vi "Load Instrument Classes.vi"(8 "error in (no error)":errorcluster, 11 "Control Experiment":refnum<class "SMO.Control Experiment.lvclass">) -> (0 "error out":errorcluster, 3 "Control Experiment out":refnum<class "SMO.Control Experiment.lvclass">)   [LabVIEW 2019, in "SMO.Control Experiment.lvclass"]
uses:
  SMO.Control Experiment.lvclass
  SMO.Control Experiment.lvclass/SMO.Control Experiment.ctl
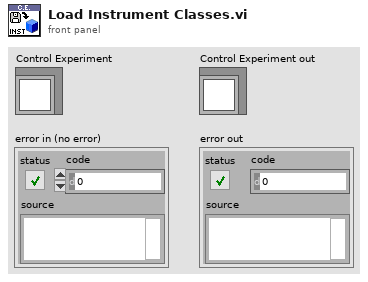
[diagram p1: front panel]
types:
  T1 = typedef "SMO.Control Experiment.lvclass/Instrument--enum.ctl" = enum16{"----- AFM/EBL -----", "AGILENT", "CYPHER", "Gemini2", "JEOL", "MFP3D", "----- Cryostat -----", "CF900", "DR200", "MNK", "PPMS 1", "PPMS 2", "PPMS 3", "----- Optics -----", "THz 1", "THz 2"}
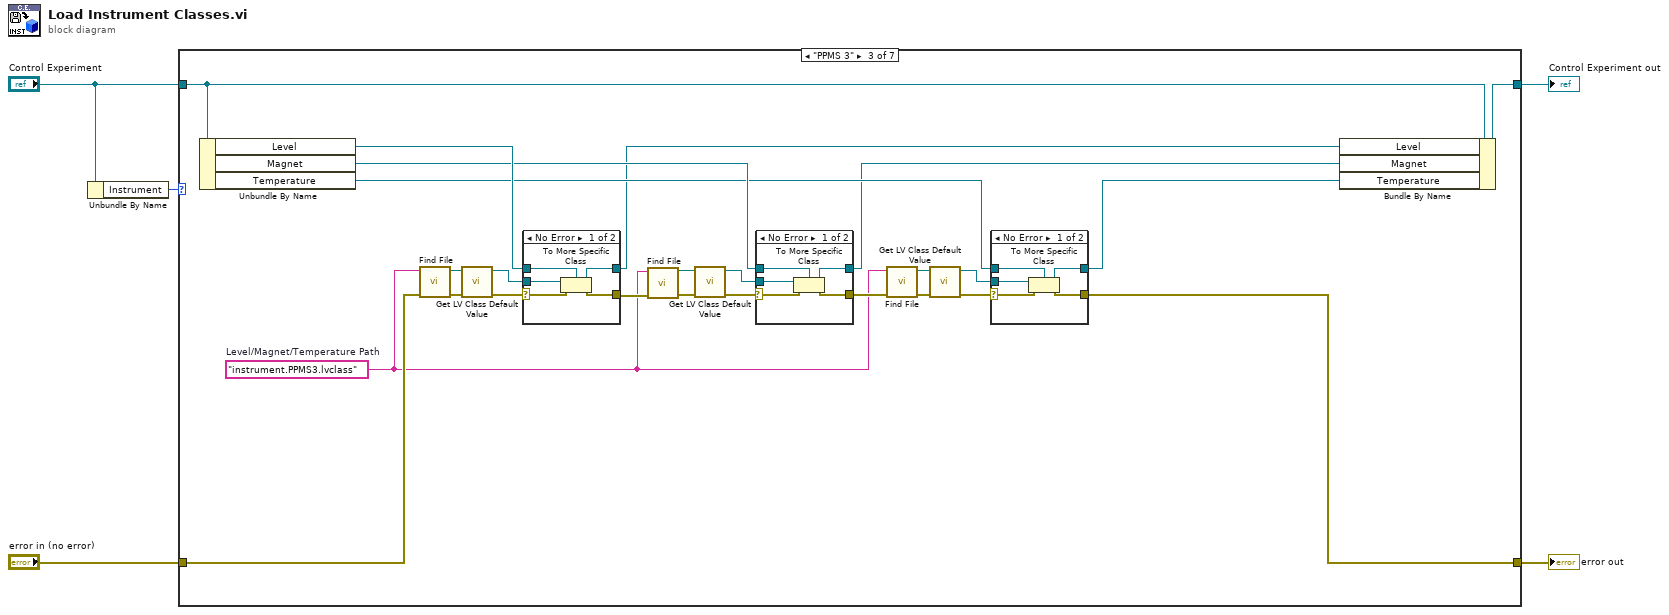
[diagram p0: block diagram]
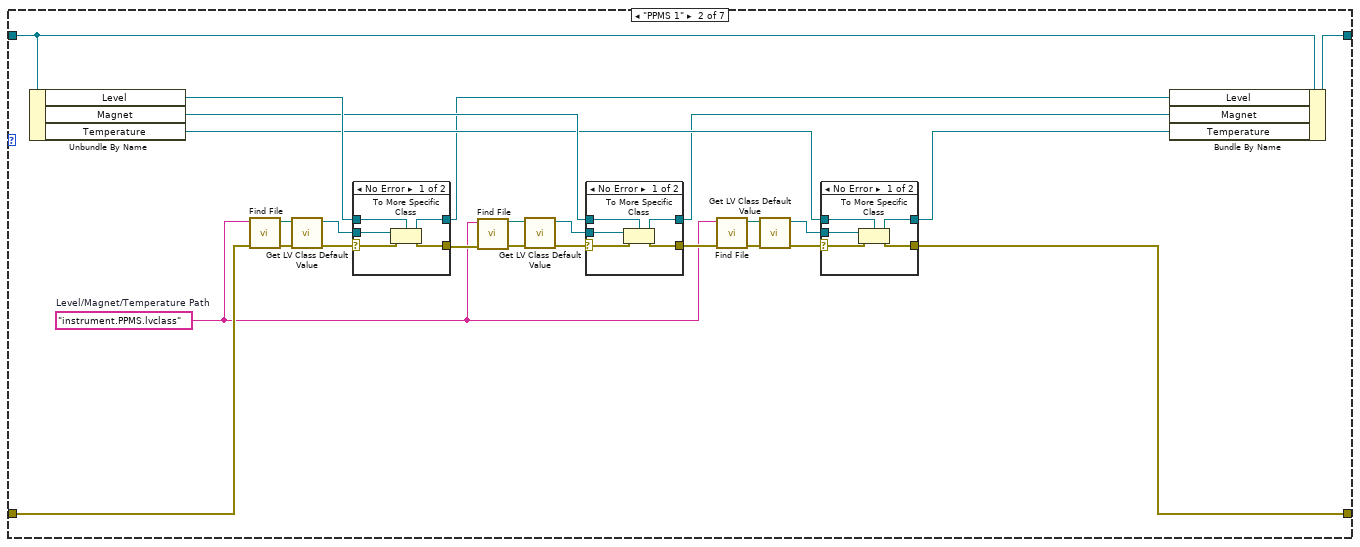
[diagram p3: hidden frame]
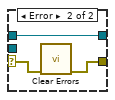
[diagram p4: hidden frame]
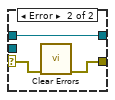
[diagram p5: hidden frame]
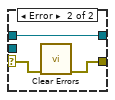
[diagram p6: hidden frame]
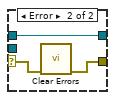
[diagram p7: hidden frame]
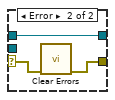
[diagram p8: hidden frame]
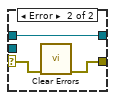
[diagram p9: hidden frame]
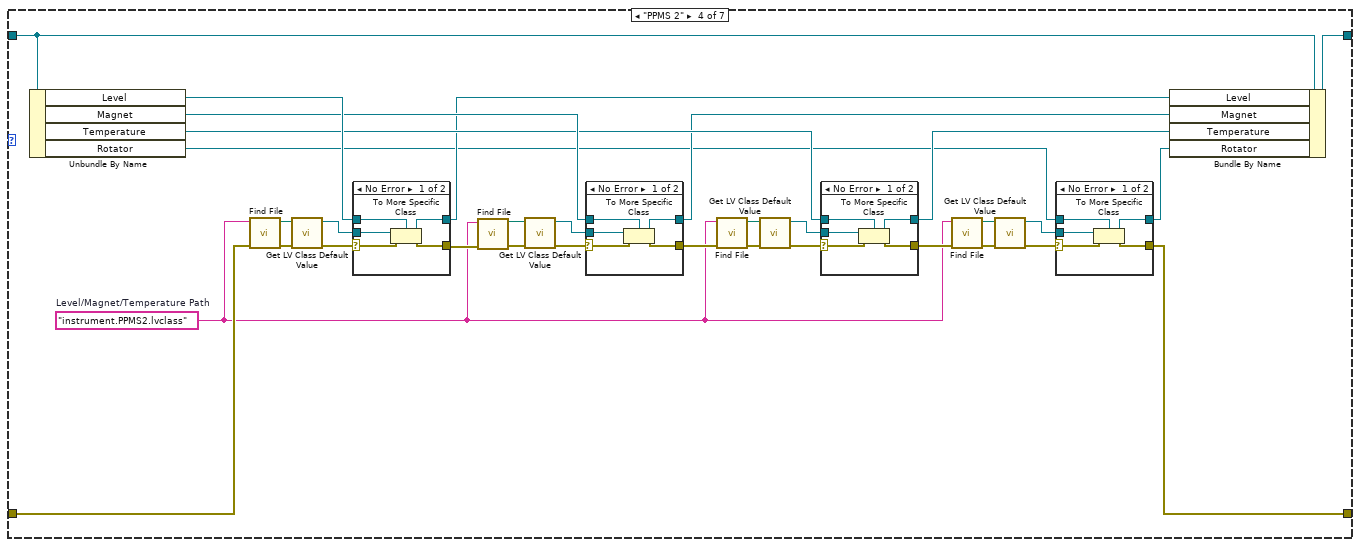
[diagram p10: hidden frame]
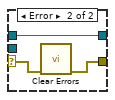
[diagram p11: hidden frame]
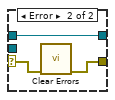
[diagram p12: hidden frame]
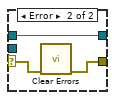
[diagram p13: hidden frame]
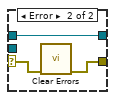
[diagram p14: hidden frame]
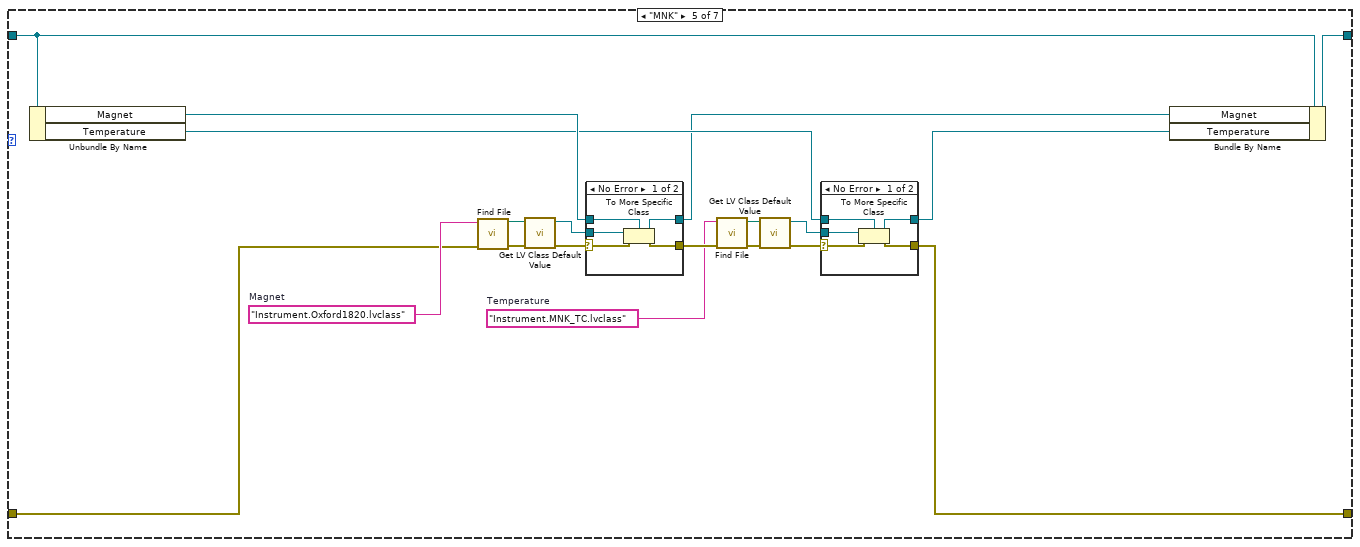
[diagram p15: hidden frame]
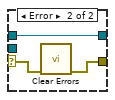
[diagram p16: hidden frame]
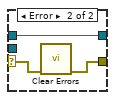
[diagram p17: hidden frame]
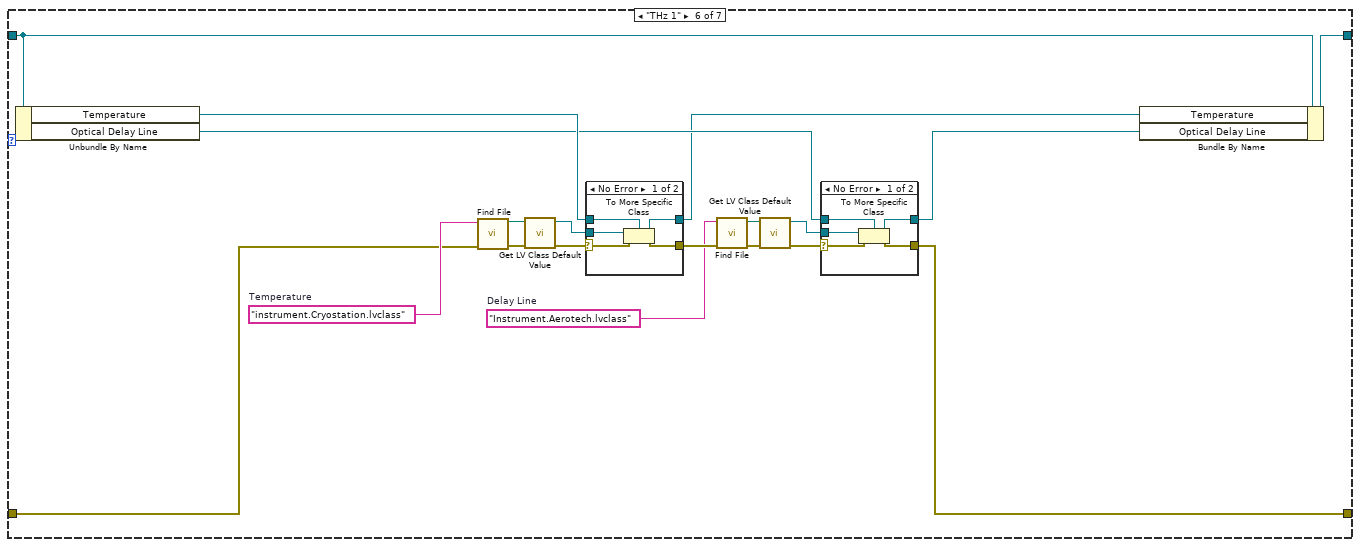
[diagram p18: hidden frame]
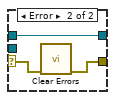
[diagram p19: hidden frame]
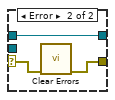
[diagram p20: hidden frame]
diagram:
  n1 = Unbundle By Name("Control Experiment") -> ("Instrument"=w2:T1)
  n2 = case shown="\"PPMS 3\"" w2 {
    tunnel: [w6 w18 w67 w107 w170 w205 w240] -> w5
    tunnel: [w7 w32 w81 w137 w188 w223 w266] -> w4
    tunnel: "Control Experiment" -> [w7 w31 w80 w136 w187 w222 w265]
    tunnel: "error in (no error)" -> [w6 w17 w66 w123 w171 w206 w257]
    frame Default {
    }
    frame "PPMS 1" {
      w8 = "instrument.PPMS.lvclass"  # Level/Magnet/Temperature Path
      n3 = Unbundle By Name(w31) -> ("Level"=w28:refnum<class "Instrument.Cryostat.lvclass">, "Magnet"=w23:refnum<class "Instrument.Cryostat.lvclass">, "Temperature"=w22:refnum<class "Instrument.Cryostat.lvclass">)
      n4 = call "Find File.vi"("error in (no error)"=w17, "File Name"=w8) -> ("error out"=w19:errorcluster, "Path"=w15:path)  [unwired: 8 in]
      n5 = call <vilib>:"Get LV Class Default Value.vi"("error in (no error)"=w19, "class path"=w15) -> ("error out"=w29:errorcluster, "object"=w30:refnum<class>)  [unwired: 8 in]
      n6 = case shown="No Error" w29 {
        selector: w29 -> [w43 w46]
        tunnel: [w41 w47] -> w16
        tunnel: w30 -> [w45 _]
        tunnel: [w44 w48] -> w12
        tunnel: w28 -> [w42 w47]
        frame No Error {
          n7 = To More Specific Class(target class=w42, reference=w45, error in=w43) -> (specific class reference=w41:refnum<class "Instrument.Cryostat.lvclass">, error out=w44:errorcluster)
        }
        frame Error {
          n8 = call <vilib>:"Clear Errors.vi"("error in (no error)"=w46) -> ("error out"=w48:errorcluster)  [unwired: 5 in, 1 out]
        }
      }
      n9 = call "Find File.vi"("error in (no error)"=w12, "File Name"=w8) -> ("error out"=w14:errorcluster, "Path"=w13:path)  [unwired: 8 in]
      n10 = call <vilib>:"Get LV Class Default Value.vi"("error in (no error)"=w14, "class path"=w13) -> ("error out"=w27:errorcluster, "object"=w26:refnum<class>)  [unwired: 8 in]
      n11 = case shown="No Error" w27 {
        selector: w27 -> [w35 w38]
        tunnel: [w33 w39] -> w20
        tunnel: w26 -> [w37 _]
        tunnel: [w36 w40] -> w9
        tunnel: w23 -> [w34 w39]
        frame No Error {
          n12 = To More Specific Class(target class=w34, reference=w37, error in=w35) -> (specific class reference=w33:refnum<class "Instrument.Cryostat.lvclass">, error out=w36:errorcluster)
        }
        frame Error {
          n13 = call <vilib>:"Clear Errors.vi"("error in (no error)"=w38) -> ("error out"=w40:errorcluster)  [unwired: 5 in, 1 out]
        }
      }
      n14 = call "Find File.vi"("error in (no error)"=w9, "File Name"=w8) -> ("error out"=w11:errorcluster, "Path"=w10:path)  [unwired: 8 in]
      n15 = call <vilib>:"Get LV Class Default Value.vi"("error in (no error)"=w11, "class path"=w10) -> ("error out"=w24:errorcluster, "object"=w25:refnum<class>)  [unwired: 8 in]
      n16 = case shown="No Error" w24 {
        selector: w24 -> [w51 w54]
        tunnel: [w49 w55] -> w21
        tunnel: w25 -> [w53 _]
        tunnel: [w52 w56] -> w18
        tunnel: w22 -> [w50 w55]
        frame No Error {
          n17 = To More Specific Class(target class=w50, reference=w53, error in=w51) -> (specific class reference=w49:refnum<class "Instrument.Cryostat.lvclass">, error out=w52:errorcluster)
        }
        frame Error {
          n18 = call <vilib>:"Clear Errors.vi"("error in (no error)"=w54) -> ("error out"=w56:errorcluster)  [unwired: 5 in, 1 out]
        }
      }
      n19 = Bundle By Name(cluster=w31, "Level"=w16, "Magnet"=w20, "Temperature"=w21) -> (w32:refnum<class "SMO.Control Experiment.lvclass">)
    }
    frame "PPMS 3" {
      w57 = "instrument.PPMS3.lvclass"  # Level/Magnet/Temperature Path
      n20 = Unbundle By Name(w80) -> ("Level"=w77:refnum<class "Instrument.Cryostat.lvclass">, "Magnet"=w72:refnum<class "Instrument.Cryostat.lvclass">, "Temperature"=w71:refnum<class "Instrument.Cryostat.lvclass">)
      n21 = call "Find File.vi"("error in (no error)"=w66, "File Name"=w57) -> ("error out"=w68:errorcluster, "Path"=w64:path)  [unwired: 8 in]
      n22 = call <vilib>:"Get LV Class Default Value.vi"("error in (no error)"=w68, "class path"=w64) -> ("error out"=w78:errorcluster, "object"=w79:refnum<class>)  [unwired: 8 in]
      n23 = case shown="No Error" w78 {
        selector: w78 -> [w92 w95]
        tunnel: [w90 w96] -> w65
        tunnel: w79 -> [w94 _]
        tunnel: [w93 w97] -> w61
        tunnel: w77 -> [w91 w96]
        frame No Error {
          n24 = To More Specific Class(target class=w91, reference=w94, error in=w92) -> (specific class reference=w90:refnum<class "Instrument.Cryostat.lvclass">, error out=w93:errorcluster)
        }
        frame Error {
          n25 = call <vilib>:"Clear Errors.vi"("error in (no error)"=w95) -> ("error out"=w97:errorcluster)  [unwired: 5 in, 1 out]
        }
      }
      n26 = call "Find File.vi"("error in (no error)"=w61, "File Name"=w57) -> ("error out"=w63:errorcluster, "Path"=w62:path)  [unwired: 8 in]
      n27 = call <vilib>:"Get LV Class Default Value.vi"("error in (no error)"=w63, "class path"=w62) -> ("error out"=w76:errorcluster, "object"=w75:refnum<class>)  [unwired: 8 in]
      n28 = case shown="No Error" w76 {
        selector: w76 -> [w84 w87]
        tunnel: [w82 w88] -> w69
        tunnel: w75 -> [w86 _]
        tunnel: [w85 w89] -> w58
        tunnel: w72 -> [w83 w88]
        frame No Error {
          n29 = To More Specific Class(target class=w83, reference=w86, error in=w84) -> (specific class reference=w82:refnum<class "Instrument.Cryostat.lvclass">, error out=w85:errorcluster)
        }
        frame Error {
          n30 = call <vilib>:"Clear Errors.vi"("error in (no error)"=w87) -> ("error out"=w89:errorcluster)  [unwired: 5 in, 1 out]
        }
      }
      n31 = call "Find File.vi"("error in (no error)"=w58, "File Name"=w57) -> ("error out"=w60:errorcluster, "Path"=w59:path)  [unwired: 8 in]
      n32 = call <vilib>:"Get LV Class Default Value.vi"("error in (no error)"=w60, "class path"=w59) -> ("error out"=w73:errorcluster, "object"=w74:refnum<class>)  [unwired: 8 in]
      n33 = case shown="No Error" w73 {
        selector: w73 -> [w100 w103]
        tunnel: [w98 w104] -> w70
        tunnel: w74 -> [w102 _]
        tunnel: [w101 w105] -> w67
        tunnel: w71 -> [w99 w104]
        frame No Error {
          n34 = To More Specific Class(target class=w99, reference=w102, error in=w100) -> (specific class reference=w98:refnum<class "Instrument.Cryostat.lvclass">, error out=w101:errorcluster)
        }
        frame Error {
          n35 = call <vilib>:"Clear Errors.vi"("error in (no error)"=w103) -> ("error out"=w105:errorcluster)  [unwired: 5 in, 1 out]
        }
      }
      n36 = Bundle By Name(cluster=w80, "Level"=w65, "Magnet"=w69, "Temperature"=w70) -> (w81:refnum<class "SMO.Control Experiment.lvclass">)
    }
    frame "PPMS 2" {
      w106 = "instrument.PPMS2.lvclass"  # Level/Magnet/Temperature Path
      n37 = Unbundle By Name(w136) -> ("Level"=w133:refnum<class "Instrument.Cryostat.lvclass">, "Magnet"=w128:refnum<class "Instrument.Cryostat.lvclass">, "Temperature"=w127:refnum<class "Instrument.Cryostat.lvclass">, "Rotator"=w109:refnum<class "Instrument.Cryostat.lvclass">)
      n38 = call "Find File.vi"("error in (no error)"=w123, "File Name"=w106) -> ("error out"=w124:errorcluster, "Path"=w121:path)  [unwired: 8 in]
      n39 = call <vilib>:"Get LV Class Default Value.vi"("error in (no error)"=w124, "class path"=w121) -> ("error out"=w134:errorcluster, "object"=w135:refnum<class>)  [unwired: 8 in]
      n40 = case shown="No Error" w134 {
        selector: w134 -> [w156 w159]
        tunnel: [w154 w160] -> w122
        tunnel: w135 -> [w158 _]
        tunnel: [w157 w161] -> w118
        tunnel: w133 -> [w155 w160]
        frame No Error {
          n41 = To More Specific Class(target class=w155, reference=w158, error in=w156) -> (specific class reference=w154:refnum<class "Instrument.Cryostat.lvclass">, error out=w157:errorcluster)
        }
        frame Error {
          n42 = call <vilib>:"Clear Errors.vi"("error in (no error)"=w159) -> ("error out"=w161:errorcluster)  [unwired: 5 in, 1 out]
        }
      }
      n43 = call "Find File.vi"("error in (no error)"=w118, "File Name"=w106) -> ("error out"=w120:errorcluster, "Path"=w119:path)  [unwired: 8 in]
      n44 = call <vilib>:"Get LV Class Default Value.vi"("error in (no error)"=w120, "class path"=w119) -> ("error out"=w132:errorcluster, "object"=w131:refnum<class>)  [unwired: 8 in]
      n45 = case shown="No Error" w132 {
        selector: w132 -> [w148 w151]
        tunnel: [w146 w152] -> w125
        tunnel: w131 -> [w150 _]
        tunnel: [w149 w153] -> w115
        tunnel: w128 -> [w147 w152]
        frame No Error {
          n46 = To More Specific Class(target class=w147, reference=w150, error in=w148) -> (specific class reference=w146:refnum<class "Instrument.Cryostat.lvclass">, error out=w149:errorcluster)
        }
        frame Error {
          n47 = call <vilib>:"Clear Errors.vi"("error in (no error)"=w151) -> ("error out"=w153:errorcluster)  [unwired: 5 in, 1 out]
        }
      }
      n48 = call "Find File.vi"("error in (no error)"=w115, "File Name"=w106) -> ("error out"=w117:errorcluster, "Path"=w116:path)  [unwired: 8 in]
      n49 = call <vilib>:"Get LV Class Default Value.vi"("error in (no error)"=w117, "class path"=w116) -> ("error out"=w129:errorcluster, "object"=w130:refnum<class>)  [unwired: 8 in]
      n50 = case shown="No Error" w129 {
        selector: w129 -> [w164 w167]
        tunnel: [w162 w168] -> w126
        tunnel: w130 -> [w166 _]
        tunnel: [w165 w169] -> w110
        tunnel: w127 -> [w163 w168]
        frame No Error {
          n51 = To More Specific Class(target class=w163, reference=w166, error in=w164) -> (specific class reference=w162:refnum<class "Instrument.Cryostat.lvclass">, error out=w165:errorcluster)
        }
        frame Error {
          n52 = call <vilib>:"Clear Errors.vi"("error in (no error)"=w167) -> ("error out"=w169:errorcluster)  [unwired: 5 in, 1 out]
        }
      }
      n53 = call "Find File.vi"("error in (no error)"=w110, "File Name"=w106) -> ("error out"=w113:errorcluster, "Path"=w114:path)  [unwired: 8 in]
      n54 = call <vilib>:"Get LV Class Default Value.vi"("error in (no error)"=w113, "class path"=w114) -> ("error out"=w112:errorcluster, "object"=w111:refnum<class>)  [unwired: 8 in]
      n55 = case shown="No Error" w112 {
        selector: w112 -> [w140 w143]
        tunnel: [w138 w144] -> w108
        tunnel: w111 -> [w142 _]
        tunnel: [w141 w145] -> w107
        tunnel: w109 -> [w139 w144]
        frame No Error {
          n56 = To More Specific Class(target class=w139, reference=w142, error in=w140) -> (specific class reference=w138:refnum<class "Instrument.Cryostat.lvclass">, error out=w141:errorcluster)
        }
        frame Error {
          n57 = call <vilib>:"Clear Errors.vi"("error in (no error)"=w143) -> ("error out"=w145:errorcluster)  [unwired: 5 in, 1 out]
        }
      }
      n58 = Bundle By Name(cluster=w136, "Level"=w122, "Magnet"=w125, "Temperature"=w126, "Rotator"=w108) -> (w137:refnum<class "SMO.Control Experiment.lvclass">)
    }
    frame "MNK" {
      w173 = "Instrument.MNK_TC.lvclass"  # Temperature
      w172 = "Instrument.Oxford1820.lvclass"  # Magnet
      n59 = Unbundle By Name(w187) -> ("Magnet"=w182:refnum<class "Instrument.Cryostat.lvclass">, "Temperature"=w181:refnum<class "Instrument.Cryostat.lvclass">)
      n60 = call "Find File.vi"("error in (no error)"=w171, "File Name"=w172) -> ("error out"=w178:errorcluster, "Path"=w177:path)  [unwired: 8 in]
      n61 = call <vilib>:"Get LV Class Default Value.vi"("error in (no error)"=w178, "class path"=w177) -> ("error out"=w186:errorcluster, "object"=w185:refnum<class>)  [unwired: 8 in]
      n62 = case shown="No Error" w186 {
        selector: w186 -> [w191 w194]
        tunnel: [w189 w195] -> w179
        tunnel: w185 -> [w193 _]
        tunnel: [w192 w196] -> w174
        tunnel: w182 -> [w190 w195]
        frame No Error {
          n63 = To More Specific Class(target class=w190, reference=w193, error in=w191) -> (specific class reference=w189:refnum<class "Instrument.Cryostat.lvclass">, error out=w192:errorcluster)
        }
        frame Error {
          n64 = call <vilib>:"Clear Errors.vi"("error in (no error)"=w194) -> ("error out"=w196:errorcluster)  [unwired: 5 in, 1 out]
        }
      }
      n65 = call "Find File.vi"("error in (no error)"=w174, "File Name"=w173) -> ("error out"=w176:errorcluster, "Path"=w175:path)  [unwired: 8 in]
      n66 = call <vilib>:"Get LV Class Default Value.vi"("error in (no error)"=w176, "class path"=w175) -> ("error out"=w183:errorcluster, "object"=w184:refnum<class>)  [unwired: 8 in]
      n67 = case shown="No Error" w183 {
        selector: w183 -> [w199 w202]
        tunnel: [w197 w203] -> w180
        tunnel: w184 -> [w201 _]
        tunnel: [w200 w204] -> w170
        tunnel: w181 -> [w198 w203]
        frame No Error {
          n68 = To More Specific Class(target class=w198, reference=w201, error in=w199) -> (specific class reference=w197:refnum<class "Instrument.Cryostat.lvclass">, error out=w200:errorcluster)
        }
        frame Error {
          n69 = call <vilib>:"Clear Errors.vi"("error in (no error)"=w202) -> ("error out"=w204:errorcluster)  [unwired: 5 in, 1 out]
        }
      }
      n70 = Bundle By Name(cluster=w187, "Magnet"=w179, "Temperature"=w180) -> (w188:refnum<class "SMO.Control Experiment.lvclass">)
    }
    frame "THz 1" {
      w208 = "Instrument.Aerotech.lvclass"  # Delay Line
      w207 = "instrument.Cryostation.lvclass"  # Temperature
      n71 = Unbundle By Name(w222) -> ("Temperature"=w217:refnum<class "Instrument.Cryostat.lvclass">, "Optical Delay Line"=w216:refnum<class "Instrument.DelayLine.lvclass">)
      n72 = call "Find File.vi"("error in (no error)"=w206, "File Name"=w207) -> ("error out"=w213:errorcluster, "Path"=w212:path)  [unwired: 8 in]
      n73 = call <vilib>:"Get LV Class Default Value.vi"("error in (no error)"=w213, "class path"=w212) -> ("error out"=w221:errorcluster, "object"=w220:refnum<class>)  [unwired: 8 in]
      n74 = case shown="No Error" w221 {
        selector: w221 -> [w226 w229]
        tunnel: [w224 w230] -> w214
        tunnel: w220 -> [w228 _]
        tunnel: [w227 w231] -> w209
        tunnel: w217 -> [w225 w230]
        frame No Error {
          n75 = To More Specific Class(target class=w225, reference=w228, error in=w226) -> (specific class reference=w224:refnum<class "Instrument.Cryostat.lvclass">, error out=w227:errorcluster)
        }
        frame Error {
          n76 = call <vilib>:"Clear Errors.vi"("error in (no error)"=w229) -> ("error out"=w231:errorcluster)  [unwired: 5 in, 1 out]
        }
      }
      n77 = call "Find File.vi"("error in (no error)"=w209, "File Name"=w208) -> ("error out"=w211:errorcluster, "Path"=w210:path)  [unwired: 8 in]
      n78 = call <vilib>:"Get LV Class Default Value.vi"("error in (no error)"=w211, "class path"=w210) -> ("error out"=w218:errorcluster, "object"=w219:refnum<class>)  [unwired: 8 in]
      n79 = case shown="No Error" w218 {
        selector: w218 -> [w234 w237]
        tunnel: [w232 w238] -> w215
        tunnel: w219 -> [w236 _]
        tunnel: [w235 w239] -> w205
        tunnel: w216 -> [w233 w238]
        frame No Error {
          n80 = To More Specific Class(target class=w233, reference=w236, error in=w234) -> (specific class reference=w232:refnum<class "Instrument.DelayLine.lvclass">, error out=w235:errorcluster)
        }
        frame Error {
          n81 = call <vilib>:"Clear Errors.vi"("error in (no error)"=w237) -> ("error out"=w239:errorcluster)  [unwired: 5 in, 1 out]
        }
      }
      n82 = Bundle By Name(cluster=w222, "Temperature"=w214, "Optical Delay Line"=w215) -> (w223:refnum<class "SMO.Control Experiment.lvclass">)
    }
    frame "DR200" {
      w243 = "RP100.lvclass"  # Strain
      w251 = "AH2500A.lvclass"  # Bridge
      w258 = "IPS120.lvclass"  # Magnet
      n83 = Unbundle By Name(w265) -> ("Magnet"=w262:refnum<class "Instrument.Cryostat.lvclass">, "C Bridge"=w249:refnum<class "Instrument.CBridge.lvclass">, "Strain Cell"=w242:refnum<class "Instrument.Strain.lvclass">)
      n84 = call "Find File.vi"("error in (no error)"=w257, "File Name"=w258) -> ("error out"=w260:errorcluster, "Path"=w259:path)  [unwired: 8 in]
      n85 = call <vilib>:"Get LV Class Default Value.vi"("error in (no error)"=w260, "class path"=w259) -> ("error out"=w264:errorcluster, "object"=w263:refnum<class>)  [unwired: 8 in]
      n86 = case shown="No Error" w264 {
        selector: w264 -> [w285 w288]
        tunnel: [w283 w289] -> w261
        tunnel: w263 -> [w287 _]
        tunnel: [w286 w290] -> w252
        tunnel: w262 -> [w284 w289]
        frame No Error {
          n87 = To More Specific Class(target class=w284, reference=w287, error in=w285) -> (specific class reference=w283:refnum<class "Instrument.Cryostat.lvclass">, error out=w286:errorcluster)
        }
        frame Error {
          n88 = call <vilib>:"Clear Errors.vi"("error in (no error)"=w288) -> ("error out"=w290:errorcluster)  [unwired: 5 in, 1 out]
        }
      }
      n89 = call "Find File.vi"("error in (no error)"=w252, "File Name"=w251) -> ("error out"=w255:errorcluster, "Path"=w256:path)  [unwired: 8 in]
      n90 = call <vilib>:"Get LV Class Default Value.vi"("error in (no error)"=w255, "class path"=w256) -> ("error out"=w253:errorcluster, "object"=w254:refnum<class>)  [unwired: 8 in]
      n91 = case shown="No Error" w253 {
        selector: w253 -> [w277 w280]
        tunnel: [w275 w281] -> w250
        tunnel: w254 -> [w279 _]
        tunnel: [w278 w282] -> w244
        tunnel: w249 -> [w276 w281]
        frame No Error {
          n92 = To More Specific Class(target class=w276, reference=w279, error in=w277) -> (specific class reference=w275:refnum<class "Instrument.CBridge.lvclass">, error out=w278:errorcluster)
        }
        frame Error {
          n93 = call <vilib>:"Clear Errors.vi"("error in (no error)"=w280) -> ("error out"=w282:errorcluster)  [unwired: 5 in, 1 out]
        }
      }
      n94 = call "Find File.vi"("error in (no error)"=w244, "File Name"=w243) -> ("error out"=w246:errorcluster, "Path"=w245:path)  [unwired: 8 in]
      n95 = call <vilib>:"Get LV Class Default Value.vi"("error in (no error)"=w246, "class path"=w245) -> ("error out"=w248:errorcluster, "object"=w247:refnum<class>)  [unwired: 8 in]
      n96 = case shown="No Error" w248 {
        selector: w248 -> [w269 w272]
        tunnel: [w267 w273] -> w241
        tunnel: w247 -> [w271 _]
        tunnel: [w270 w274] -> w240
        tunnel: w242 -> [w268 w273]
        frame No Error {
          n97 = To More Specific Class(target class=w268, reference=w271, error in=w269) -> (specific class reference=w267:refnum<class "Instrument.Strain.lvclass">, error out=w270:errorcluster)
        }
        frame Error {
          n98 = call <vilib>:"Clear Errors.vi"("error in (no error)"=w272) -> ("error out"=w274:errorcluster)  [unwired: 5 in, 1 out]
        }
      }
      n99 = Bundle By Name(cluster=w265, "Magnet"=w261, "C Bridge"=w250, "Strain Cell"=w241) -> (w266:refnum<class "SMO.Control Experiment.lvclass">)
    }
  }
  "error out" <- w5
  "Control Experiment out" <- w4
